vi "First step initialization (SILAR).vi"(7 "COM порт":refnum<visa-resource-name>) -> (0 "Error Out":errorcluster, 3 "Arduino Resource Out":T1={"VISA resource"="", "Board Type"=enum."Uno", "Connection Type"=enum."USB / Serial", "Bytes Per Packet (15)"=15})   [LabVIEW 2016]
uses:
  <vilib>/LabVIEW Interface for Arduino/Type Defs/Arduino Resource.ctl
  <vilib>/LabVIEW Interface for Arduino/Type Defs/Board Type.ctl
  <vilib>/LabVIEW Interface for Arduino/LabVIEW Interface for Arduino.lvlib
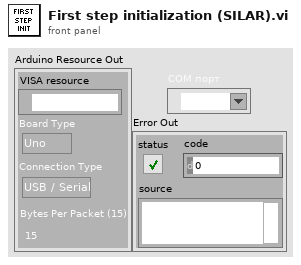
[diagram p1: front panel]
types:
  T1 = typedef "LabVIEW Interface for Arduino.lvlib/Arduino Resource.ctl" = cluster{"VISA resource":refnum<visa-resource-name>, "Board Type":T2, "Connection Type":enum8{"USB / Serial"}, "Bytes Per Packet (15)":u8}
  T2 = typedef "LabVIEW Interface for Arduino.lvlib/Board Type.ctl" = enum16{"Uno", "Dimuelanove w/Atmega 328", "Mega 2560"}
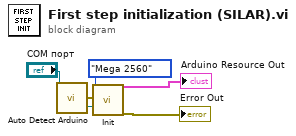
[diagram p0: block diagram]
diagram:
  n1 = call <vilib>:"Auto Detect Arduino.vi"("Visa Resource"="COM порт") -> ("VISA resource"=w6:refnum<visa-resource-name>, "error out"=w5:errorcluster)  [unwired: 13 in]
  n2 = call <vilib>:"Init.vi"("VISA resource"=w6, "Board Type (Uno)"=Board_Type."Mega 2560", "error in"=w5) -> ("Arduino Resource"=→"Arduino Resource Out":T1, "error out"=→"Error Out":errorcluster)  [unwired: 15 in]
